vi "FSM Seal.vi"(0 "Signals":T5, 1 "Test and Offset Controls":T6, 2 "Holding Potential Controls":T4, 3 "Pressure Controls":T3, 4 "Autotune Gain":T2, 5 "error in (no error)":errorcluster, 6 "Seal Dynamics":T1, 7 "Capacitance Compensation":refnum<vi>, 8 "Test Signal Levels":refnum<vi>, 11 "Dialog Indicator":refnum<vi>, 13 "Abort":refnum<vi>) -> (15 "Aborted":bool, 19 "error out":errorcluster)   [LabVIEW 2012, in "Autopatcher Daemon.lvlib"]
uses:
  Autopatcher Daemon.lvlib
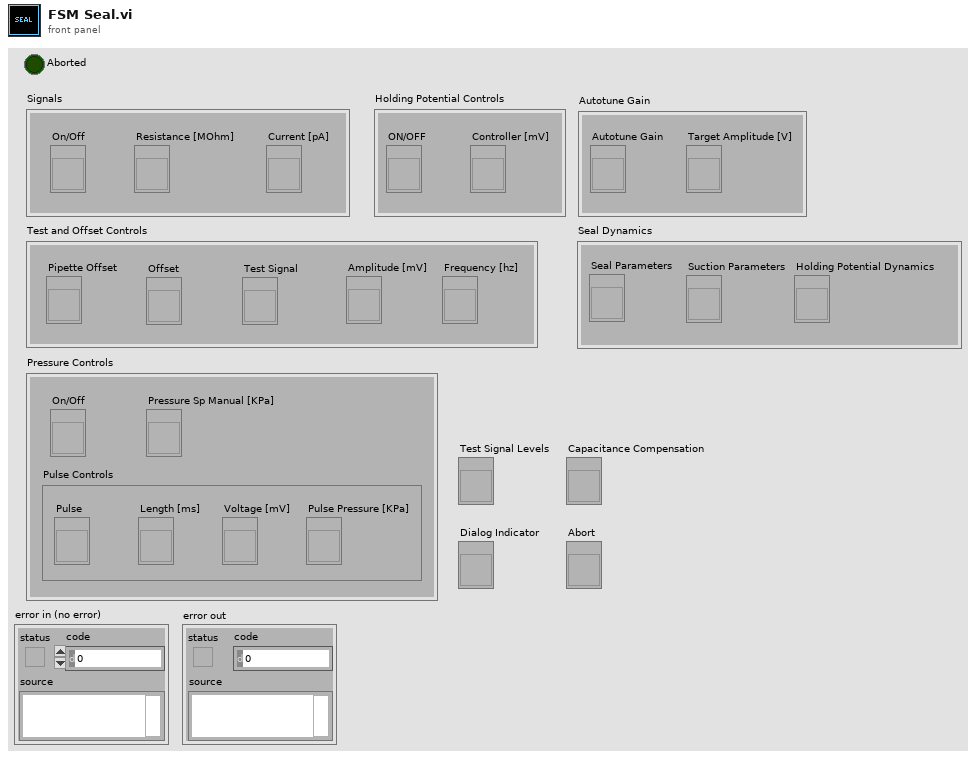
[diagram p1: front panel]
types:
  T1 = cluster{"Suction Parameters":refnum<vi>, "Holding Potential Dynamics":refnum<vi>, "Seal Parameters":refnum<vi>}
  T2 = cluster{"Autotune Gain":refnum<vi>, "Target Amplitude [V]":refnum<vi>}
  T3 = cluster{"On/Off":refnum<vi>, "Pulse Controls":cluster{"Pulse":refnum<vi>, "Length [ms]":refnum<vi>, "Voltage [mV]":refnum<vi>, "Pulse Pressure [KPa]":refnum<vi>}, "Pressure Sp Manual [KPa]":refnum<vi>}
  T4 = cluster{"ON/OFF":refnum<vi>, "Controller [mV]":refnum<vi>}
  T5 = cluster{"On/Off":refnum<vi>, "Resistance [MOhm]":refnum<vi>, "Current [pA]":refnum<vi>}
  T6 = cluster{"Pipette Offset":refnum<vi>, "Offset":refnum<vi>, "Test Signal":refnum<vi>, "Amplitude [mV]":refnum<vi>, "Frequency [hz]":refnum<vi>}
  T7 = cluster{"Start [mV]":dbl, "Target [mV]":dbl, "Speed [mV/s]":dbl}
  T8 = cluster{"Seal Target [MOhm]":dbl, "Stability Threhsold [%]":dbl, "Seal Timeout [s]":dbl, "Stability Refresh [ms]":dbl}
  T9 = cluster{"Seal":cluster{"Amplitude [mV]":i32, "Frequency [hz]":u16}, "Extracellular":cluster{"Amplitude [mV]":i32, "Frequency [hz]":u16}}
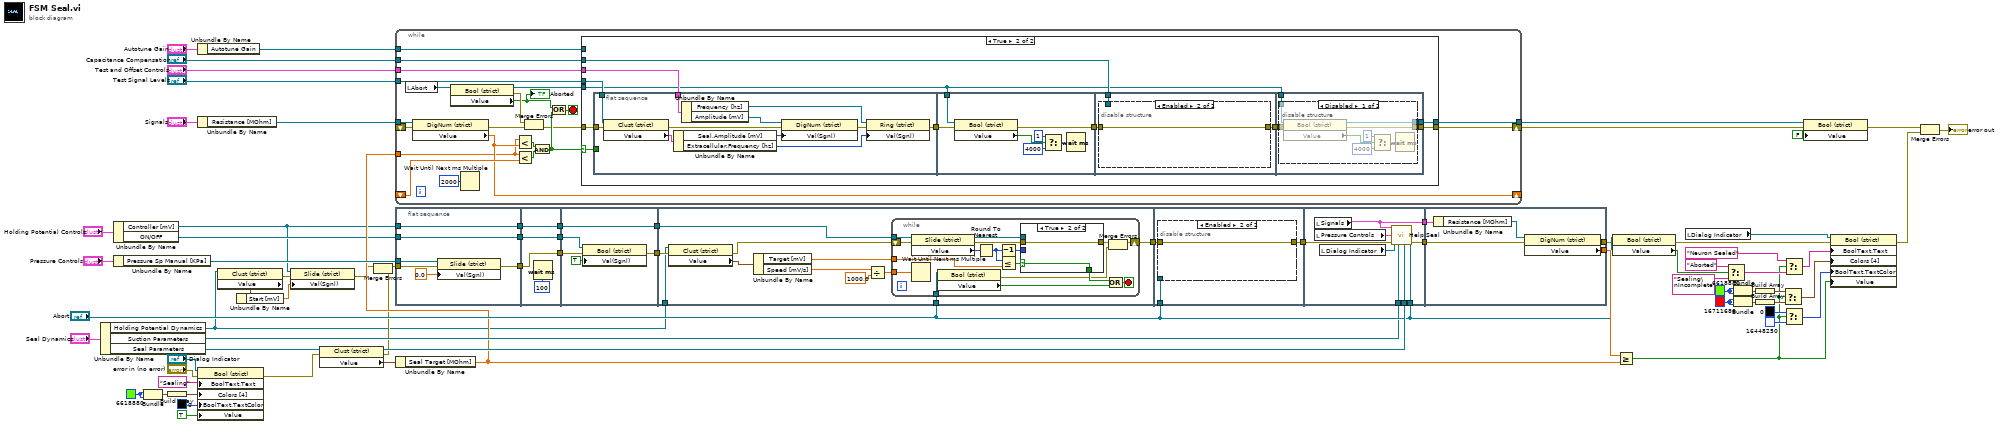
[diagram p0: block diagram]
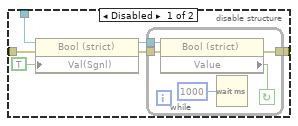
[diagram p3: hidden frame]
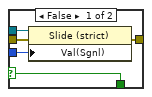
[diagram p5: hidden frame]
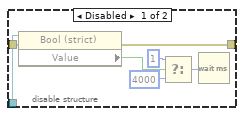
[diagram p6: hidden frame]
diagram:
  w51 = u32 6618880
  w45 = u32 16711680
  w62 = u32 6618880
  n1 = Unbundle By Name("Seal Dynamics") -> ("Holding Potential Dynamics"=w4:refnum<vi>, "Suction Parameters"=w26:refnum<vi>, "Seal Parameters"=w27:refnum<vi>)
  n2 = Unbundle By Name("Holding Potential Controls") -> ("Controller [mV]"=w2:refnum<vi>, "ON/OFF"=w3:refnum<vi>)
  n3 = Unbundle By Name("Pressure Controls") -> ("Pressure Sp Manual [KPa]"=w24:refnum<vi>)
  n4 = Bundle(w62, w62) -> (w63:cluster{u32, u32})  [unwired: 1 in]
  n5 = Build Array(w63) -> (w60:cluster{u32, u32}[])
  n6 = Unbundle By Name("Autotune Gain") -> ("Autotune Gain"=w28:refnum<vi>)
  n7 = Unbundle By Name("Signals") -> ("Resistance [MOhm]"=w71:refnum<vi>)
  n8 = property class="Bool (strict)"(reference="Dialog Indicator", error in="error in (no error)", "BoolText.Text"="Sealing" ("Boolean Text.Text"), "Colors [4]"=w60, "BoolText.TextColor"=u32 0, "Value"=TRUE) -> (error out=w57:errorcluster)  [unwired: 1 out]
  n9 = property class="Clust (strict)"(reference=w4) -> (error out=w12:errorcluster, "Value"=w11:T7)  [unwired: 1 in, 1 out]
  n10 = Unbundle By Name(w11) -> ("Start [mV]"=w10:dbl)
  n11 = property class="Slide (strict)"(reference=w2, error in=w12, "Val(Sgnl)"=w10) -> (error out=w14:errorcluster)  [unwired: 1 out]
  n12 = property class="Clust (strict)"(reference=w27, error in=w57) -> (reference out=w69:refnum<vi>, error out=w15:errorcluster, "Value"=w70:T8)
  n13 = Merge Errors(w14, w15) -> (w13:errorcluster)
  n14 = Unbundle By Name(w70) -> ("Seal Target [MOhm]"=w16:dbl)
  n15 = while {
    shift-right: [w91] -> _
    shift-left: _ -> [w96]
    tunnel: w28 -> [w92]
    tunnel: w71 -> [w90]
    tunnel: "Test Signal Levels" -> [w89]
    tunnel: "Capacitance Compensation" -> [w88]
    shift-right: [w87] -> w19
    shift-left: _ -> [w75]
    tunnel: "Test and Offset Controls" -> [w86]
    tunnel: [w78] -> w17
    tunnel: w16 -> [w76]
    stop <- w85 stop-if-true
    n16 = local read "Abort"() -> (w79:refnum<vi>)
    n17 = property class="DigNum (strict)"(reference=w90, error in=w75) -> (error out=w82:errorcluster, "Value"=w91:dbl)  [unwired: 1 out]
    n18 = property class="Bool (strict)"(reference=w79) -> (reference out=w80:refnum<vi>, error out=w81:errorcluster, "Value"=w77:bool)  [unwired: 1 in]
    "Aborted" <- w77
    n19 = Wait Until Next ms Multiple(millisecond multiple=u32 2000) -> ()  [unwired: 1 out]
    n20 = Less?(x=w76, y=w91) -> (x < y?=w95:bool)
    n21 = Less?(x=w76, y=w96) -> (x < y?=w94:bool)
    n22 = Merge Errors(w81, w82) -> (w83:errorcluster)
    n23 = And(x=w95, y=w94) -> (x .and. y?=w84:bool)
    n24 = Or(x=w77, y=w84) -> (x .or. y?=w85:bool)
    n25 = case shown="True" w84 {
      selector: w84 -> [_ w104]
      tunnel: [w98 w108] -> w87
      tunnel: w83 -> [w98 w107]
      tunnel: w92 -> [_ _]
      tunnel: w89 -> [_ w106]
      tunnel: w88 -> [_ w105]
      tunnel: w86 -> [_ w102]
      tunnel: w80 -> [w97 w101]
      tunnel: [w97 w100] -> w78
      frame False {
      }
      frame True {
        n26 = flat-sequence {
          tunnel: w104 -> [_]
          tunnel: w107 -> [w120]
          tunnel: w106 -> [w119]
          tunnel: [w113] -> w103
          tunnel: w102 -> [w111]
          tunnel: [w123] -> w109
          tunnel: w103 -> [w124]
          tunnel: w101 -> [w122]
          tunnel: w109 -> [w130]
          tunnel: w105 -> [w129]
          tunnel: [w128] -> w99
          tunnel: [w146] -> w108
          tunnel: w101 -> [w145]
          tunnel: [w144] -> w100
          tunnel: w99 -> [w143]
          frame #0 {
            n27 = property class="Clust (strict)"(reference=w119, error in=w120) -> (error out=w112:errorcluster, "Value"=w110:T9)  [unwired: 1 out]
            n28 = Unbundle By Name(w110) -> ("Seal.Amplitude [mV]"=w115:i32, "Extracellular.Frequency [hz]"=w114:u16)
            n29 = Unbundle By Name(w111) -> ("Frequency [hz]"=w117:refnum<vi>, "Amplitude [mV]"=w116:refnum<vi>)
            n30 = property class="DigNum (strict)"(reference=w116, error in=w112, "Val(Sgnl)"=w115) -> (error out=w118:errorcluster)  [unwired: 1 out]
            n31 = property class="Ring (strict)"(reference=w117, error in=w118, "Val(Sgnl)"=w114) -> (error out=w113:errorcluster)  [unwired: 1 out]
          }
          frame #1 {
            n32 = property class="Bool (strict)"(reference=w122, error in=w124) -> (error out=w123:errorcluster, "Value"=w121:bool)  [unwired: 1 out]
            n33 = Select(t=u32 1 ("milliseconds to wait"), s=w121, f=u32 4000 ("milliseconds to wait")) -> (s? t:f=w125:u32)
            n34 = Wait (ms)(milliseconds to wait=w125) -> ()  [unwired: 1 out]
          }
          frame #2 {
            n35 = disable-structure shown="Enabled" {
              disable-tunnel: w130 -> [w136 w142]
              disable-tunnel: w129 -> [w135 _]
              disable-tunnel: [w132 w142] -> w128
              frame Disabled {
                n36 = property class="Bool (strict)"(reference=w135, error in=w136, "Val(Sgnl)"=TRUE ("Value (Signaling)")) -> (reference out=w131:refnum<vi>, error out=w133:errorcluster)
                n37 = while {
                  tunnel: w133 -> [w139]
                  tunnel: [w138] -> w132
                  tunnel: w131 -> [w137]
                  stop <- w141 continue-if-true
                  n38 = property class="Bool (strict)"(reference=w137, error in=w139) -> (error out=w138:errorcluster, "Value"=w141:bool)  [unwired: 1 out]
                  n39 = Wait (ms)(milliseconds to wait=u32 1000) -> ()  [unwired: 1 out]
                }
              }
              frame Enabled {
              }
            }
          }
          frame #3 {
            n40 = disable-structure shown="Disabled" {
              disable-tunnel: [w149 w155] -> w146
              disable-tunnel: w145 -> [w148 w154]
              disable-tunnel: [w147 w154] -> w144
              disable-tunnel: w143 -> [_ w155]
              frame Disabled {
                n41 = property class="Bool (strict)"(reference=w148) -> (reference out=w147:refnum<vi>, error out=w149:errorcluster, "Value"=w153:bool)  [unwired: 1 in]
                n42 = Select(t=u32 1 ("milliseconds to wait"), s=w153, f=u32 4000 ("milliseconds to wait")) -> (s? t:f=w152:u32)
                n43 = Wait (ms)(milliseconds to wait=w152) -> ()  [unwired: 1 out]
              }
              frame Enabled {
              }
            }
          }
        }
      }
    }
  }
  n44 = flat-sequence {
    tunnel: w13 -> [w159]
    tunnel: [w158] -> w72
    tunnel: w24 -> [w160]
    tunnel: w3 -> [w157]
    tunnel: [w157] -> w67
    tunnel: [w156] -> w66
    tunnel: w2 -> [w156]
    tunnel: w72 -> [w165]
    tunnel: [w165] -> w9
    tunnel: w67 -> [w164]
    tunnel: [w164] -> w7
    tunnel: [w163] -> w6
    tunnel: w66 -> [w163]
    tunnel: w9 -> [w168]
    tunnel: [w167] -> w8
    tunnel: w7 -> [w166]
    tunnel: w6 -> [w170]
    tunnel: [w170] -> w5
    tunnel: w8 -> [w181]
    tunnel: w5 -> [w173]
    tunnel: [w179] -> w65
    tunnel: "Abort" -> [w176]
    tunnel: w4 -> [w175]
    tunnel: w65 -> [w208]
    tunnel: [w207] -> w64
    tunnel: "Abort" -> [w206]
    tunnel: [w224] -> w74
    tunnel: w69 -> [w221]
    tunnel: "Abort" -> [w222]
    tunnel: w64 -> [w223]
    tunnel: w26 -> [w220]
    tunnel: [w218] -> w23
    tunnel: w74 -> [w229]
    tunnel: [w227] -> w38
    tunnel: [w228] -> w1
    tunnel: w23 -> [w226]
    frame #0 {
      n45 = property class="Slide (strict)"(reference=w160, error in=w159, "Val(Sgnl)"=0.0 ("Pressure Set Point")) -> (error out=w158:errorcluster)  [unwired: 1 out]
    }
    frame #1 {
      n46 = Wait (ms)(milliseconds to wait=u32 100) -> ()  [unwired: 1 out]
    }
    frame #2 {
      n47 = property class="Bool (strict)"(reference=w166, error in=w168, "Val(Sgnl)"=TRUE ("Value (Signaling)")) -> (error out=w167:errorcluster)  [unwired: 1 out]
    }
    frame #3 {
      n48 = property class="Clust (strict)"(reference=w175, error in=w181) -> (error out=w174:errorcluster, "Value"=w180:T7)  [unwired: 1 out]
      n49 = Unbundle By Name(w180) -> ("Target [mV]"=w178:dbl, "Speed [mV/s]"=w172:dbl)
      n50 = Divide(x=w172, y=1000.0) -> (x/y=w177:dbl)
      n51 = while {
        tunnel: w178 -> [w196]
        tunnel: w173 -> [w195]
        shift-right: [w182] -> w179
        shift-left: w174 -> [w190]
        tunnel: w177 -> [w189]
        tunnel: w176 -> [w185]
        stop <- w186 stop-if-true
        n52 = property class="Slide (strict)"(reference=w195, error in=w190) -> (reference out=w191:refnum<vi>, error out=w193:errorcluster, "Value"=w194:i32)
        n53 = Wait Until Next ms Multiple(millisecond multiple=w189) -> ()  [unwired: 1 out]
        n54 = property class="Bool (strict)"(reference=w185) -> (error out=w184:errorcluster, "Value"=w188:bool)  [unwired: 1 in, 1 out]
        n55 = Round To Nearest(number=w194) -> (nearest integer value=w197:i32)
        n56 = Decrement(x=w197) -> (x-1=w192:i32)
        n57 = Less Or Equal?(x=w197, y=w196) -> (x <= y?=w198:bool)
        n58 = case shown="True" w198 {
          selector: w198 -> [w203 w204]
          tunnel: w193 -> [w202 w205]
          tunnel: w192 -> [w201 _]
          tunnel: [w199 w205] -> w183
          tunnel: [w203 w204] -> w187
          tunnel: w191 -> [w200 _]
          frame False {
            n59 = property class="Slide (strict)"(reference=w200, error in=w202, "Val(Sgnl)"=w201) -> (error out=w199:errorcluster)  [unwired: 1 out]
          }
          frame True {
          }
        }
        n60 = Or(x=w187, y=w188) -> (x .or. y?=w186:bool)
        n61 = Merge Errors(w183, w184) -> (w182:errorcluster)
      }
    }
    frame #4 {
      n62 = disable-structure shown="Enabled" {
        disable-tunnel: w208 -> [w211 w216]
        disable-tunnel: [w210 w216] -> w207
        disable-tunnel: w206 -> [w209 _]
        frame Disabled {
          n63 = property class="Bool (strict)"(reference=w209, error in=w211) -> (error out=w210:errorcluster, "Value"=w215:bool)  [unwired: 1 out]
          n64 = Select(t=u32 1 ("milliseconds to wait"), s=w215, f=u32 4000 ("milliseconds to wait")) -> (s? t:f=w214:u32)
          n65 = Wait (ms)(milliseconds to wait=w214) -> ()  [unwired: 1 out]
        }
        frame Enabled {
        }
      }
    }
    frame #5 {
      n66 = local read "Signals"() -> (w218:T5)
      n67 = local read "Pressure Controls"() -> (w219:T3)
      n68 = local read "Dialog Indicator"() -> (w217:refnum<vi>)
      n69 = call "Help Seal.vi"("Signals"=w218, "Pressure Controls"=w219, "Seal Parameters"=w221, "Suction Parameters"=w220, "error in (no error)"=w223, "Dialog Indicator"=w217, "Abort"=w222) -> ("error out"=w224:errorcluster)  [unwired: 7 in, 1 out]
    }
    frame #6 {
      n70 = Unbundle By Name(w226) -> ("Resistance [MOhm]"=w225:refnum<vi>)
      n71 = property class="DigNum (strict)"(reference=w225, error in=w229) -> (error out=w228:errorcluster, "Value"=w227:dbl)  [unwired: 1 out]
    }
  }
  n72 = property class="Bool (strict)"(reference="Abort", error in=w1) -> (error out=w21:errorcluster, "Value"=w39:bool)  [unwired: 1 out]
  n73 = Greater Or Equal?(x=w38, y=w16) -> (x >= y?=w40:bool)
  n74 = local read "Dialog Indicator"() -> (w34:refnum<vi>)
  n75 = Select(t="Aborted" ("Boolean Text.Text"), s=w39, f="Sealing\nIncomplete" ("Boolean Text.Text")) -> (s? t:f=w41:string)
  n76 = Bundle(w51, w51) -> (w52:cluster{u32, u32})  [unwired: 1 in]
  n77 = Bundle(w45, w45) -> (w46:cluster{u32, u32})  [unwired: 1 in]
  n78 = Build Array(w52) -> (w43:cluster{u32, u32}[])
  n79 = Build Array(w46) -> (w42:cluster{u32, u32}[])
  n80 = Select(t=w43, s=w40, f=w42) -> (s? t:f=w50:cluster{u32, u32}[])
  n81 = Select(t="Neuron Sealed" ("Boolean Text.Text"), s=w40, f=w41) -> (s? t:f=w49:string)
  n82 = Select(t=u32 0, s=w40, f=u32 16448250) -> (s? t:f=w55:u32)
  n83 = property class="Bool (strict)"(reference=w17, error in=w19, "Value"=FALSE) -> (error out=w18:errorcluster)  [unwired: 1 out]
  n84 = property class="Bool (strict)"(reference=w34, error in=w21, "BoolText.Text"=w49, "Colors [4]"=w50, "BoolText.TextColor"=w55, "Value"=w40) -> (error out=w36:errorcluster)  [unwired: 1 out]
  n85 = Merge Errors(w18, w36) -> (→"error out":errorcluster)
